vi "clicked_double_circ_trajectory.vi"(0 "ScanModeTS090821Circular2D in":refnum<class "ImagingModeTS090821Circular2D.lvclass">, 1 "clicked points":i32[][](array[numeric]), 7 "error in (no error)":errorcluster) -> (20 "ScanModeTS090821Circular2D out":refnum<class "ImagingModeTS090821Circular2D.lvclass">, 27 "error out":errorcluster)   [LabVIEW 2010, in "ImagingModeTS090821Circular2D.lvclass"]
uses:
  ImagingModeTS090821Circular2D.lvclass
  ImagingModeTS090821Circular2D.lvclass/ImagingModeTS090821Circular2D.ctl
  common/classes/Image/Image/Image.lvclass
  <vilib>/express/express arith-compare/Formula/XNode/ExpressFormulaBlockNode.xnode
  <vilib>/Analysis/BLAS.llb/dnrm2 - Vector 2-Norm (DBL).vi
  <vilib>/Analysis/NI_AALBLAS.lvlib
panel:
  out "rotation angle atan2":dbl
  out "x y centering":dbl[](array[numeric])
  out "circ_offset":dbl
  out "a amplitude":dbl
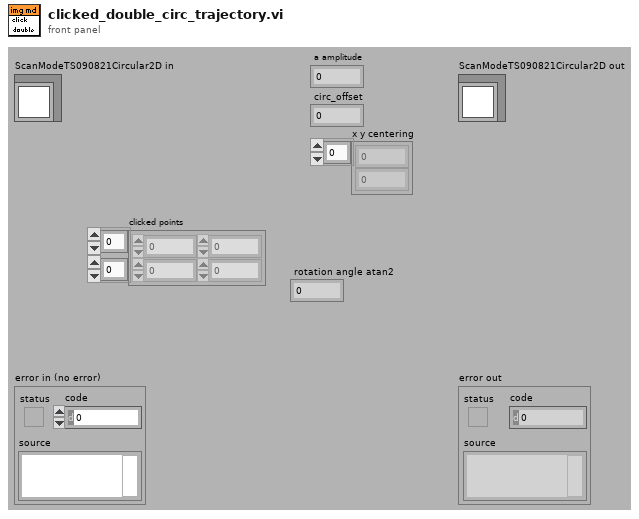
[diagram p1: front panel]
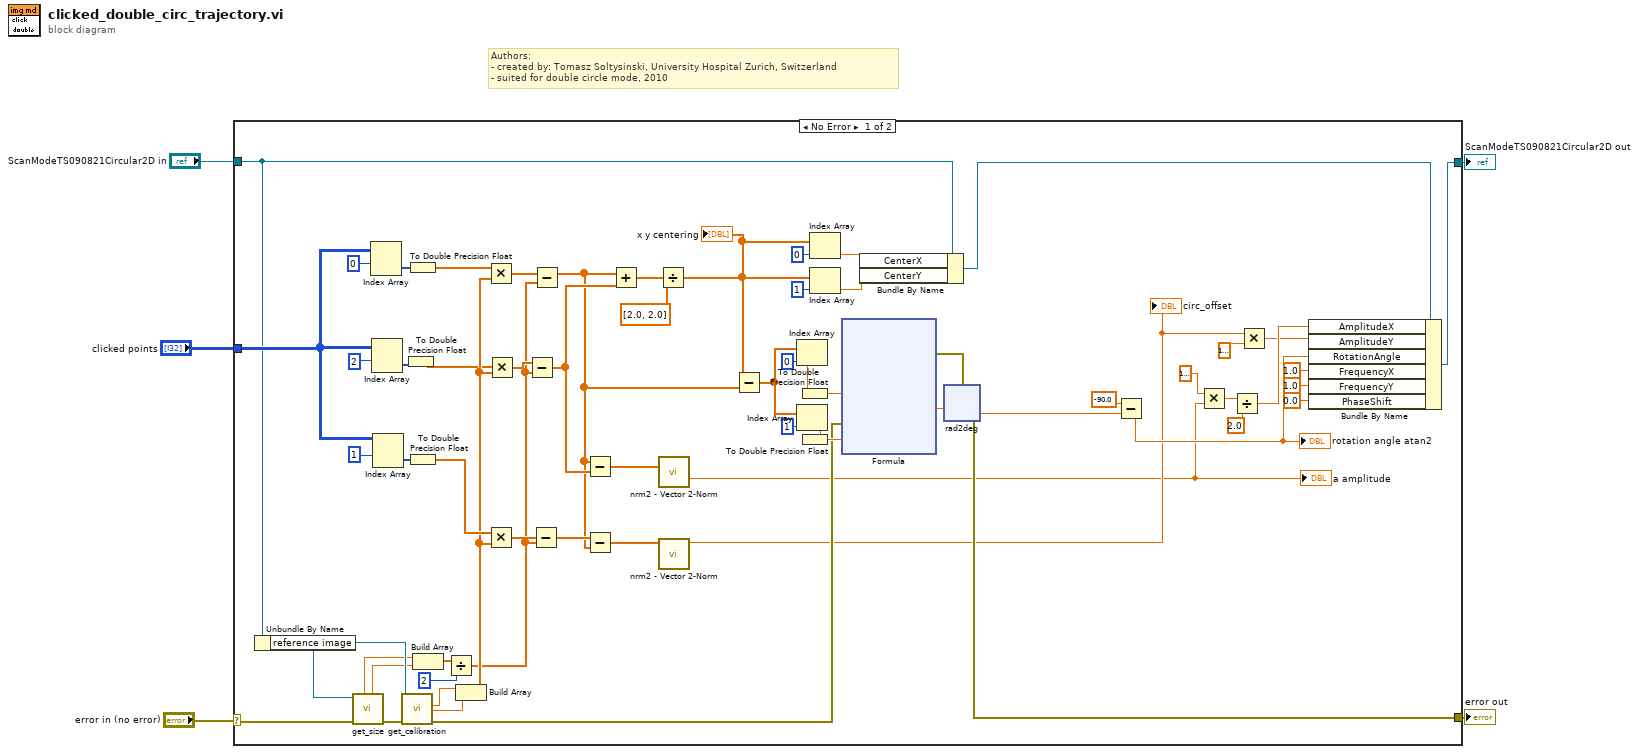
[diagram p0: block diagram]
diagram:
  # "Authors: \n- created by: Tomasz Soltysinski, University Hospital Zurich, Switzerland\n- suited for double circle mode, 2010"
  n1 = case shown="No Error" "error in (no error)" {
    selector: "error in (no error)" -> [w22 w89]
    tunnel: [w9 w89] -> w4
    tunnel: [w55 w88] -> w2
    tunnel: "ScanModeTS090821Circular2D in" -> [w26 w88]
    tunnel: "clicked points" -> [w38 _]
    frame No Error {
      n2 = Unbundle By Name(w26) -> ("reference image"=w20:refnum<class "Image.lvclass">)
      n3 = call-dynamic "get_size.vi"("error in (no error)"=w22, "Image in"=w20) -> ("error out"=w21:errorcluster, "physical size y"=w18:dbl, "physical size x"=w19:dbl)  [unwired: 2 in, 5 out]
      n4 = Index Array(array=w38, index (row)=0 ("disabled index (col)")) -> (element=w37:i32[])  [unwired: 1 in]
      n5 = Index Array(array=w38, index (row)=2 ("disabled index (col)")) -> (element=w36:i32[])  [unwired: 1 in]
      n6 = Index Array(array=w38, index (row)=1 ("disabled index (col)")) -> (element=w35:i32[])  [unwired: 1 in]
      n7 = call "get_calibration.vi"("error in (no error)"=w21, "Image.lvclass in"=w20) -> ("error out"=w25:errorcluster, "y"=w23:dbl, "x"=w24:dbl)  [unwired: 4 in, 3 out]
      n8 = To Double Precision Float(number=w36) -> (double precision float=w29:dbl[])
      n9 = To Double Precision Float(number=w37) -> (double precision float=w28:dbl[])
      n10 = To Double Precision Float(number=w35) -> (double precision float=w31:dbl[])
      n11 = Build Array(w19, w18) -> (w12:dbl[])
      n12 = Divide(x=w12, y=2 ("physical size y")) -> (x/y=w11:dbl[])
      n13 = Build Array(w24, w23) -> (w30:dbl[])
      n14 = Multiply(x=w28, y=w30) -> (x*y=w15:dbl[])
      n15 = Multiply(x=w31, y=w30) -> (x*y=w14:dbl[])
      n16 = Multiply(x=w29, y=w30) -> (x*y=w17:dbl[])
      n17 = Subtract(x=w17, y=w11) -> (x-y=w16:dbl[])
      n18 = Subtract(x=w14, y=w11) -> (x-y=w13:dbl[])
      n19 = Subtract(x=w15, y=w11) -> (x-y=w6:dbl[])
      n20 = Subtract(x=w6, y=w16) -> (x-y=w33:dbl[])
      n21 = Subtract(x=w13, y=w6) -> (x-y=w32:dbl[])
      n22 = Add(x=w6, y=w16) -> (x+y=w34:dbl[])
      n23 = Divide(x=w34, y=dbl[] [2.0, 2.0]) -> (x/y=w27:dbl[])
      "x y centering" <- w27
      n24 = call-poly <vilib>:"nrm2 - Vector 2-Norm.vi"("x"=w33) -> ("dnrm2"=w7:dbl)  [unwired: 9 in, 1 out]
      "a amplitude" <- w7
      n25 = call-poly <vilib>:"nrm2 - Vector 2-Norm.vi"("x"=w32) -> ("dnrm2"=w8:dbl)  [unwired: 9 in, 1 out]
      "circ_offset" <- w8
      n26 = Subtract(x=w27, y=w6) -> (x-y=w52:dbl[])
      n27 = Index Array(array=w52, index=0) -> (element=w51:dbl)
      n28 = Index Array(array=w52, index=1) -> (element=w49:dbl)
      n29 = To Double Precision Float(number=w51) -> (double precision float=w50:dbl)
      n30 = To Double Precision Float(number=w49) -> (double precision float=w48:dbl)
      n31 = Index Array(array=w27, index=0 ("disabled index (col)")) -> (element=w59:dbl)
      n32 = Index Array(array=w27, index=1 ("disabled index (col)")) -> (element=w57:dbl)
      n33 = xnode "Formula"("x"=w50, "error in (no error)"=w25, "y"=w48) -> ("Result"=w46:dbl, "error out"=w44:errorcluster)
      n34 = Bundle By Name(cluster=w26, "CenterX"=w59, "CenterY"=w57) -> (w56:refnum<class "ImagingModeTS090821Circular2D.lvclass">)
      n35 = xnode "rad2deg"("alfa"=w46, "error in (no error)"=w44) -> ("Result"=w45:dbl, "error out"=w9:errorcluster)
      n36 = Subtract(x=-90.0 ("y"), y=w45) -> (x-y=w39:dbl)
      "rotation angle atan2" <- w39
      n37 = Multiply(x=dbl[unit] 1e-06 ("dimension size"), y=w7) -> (x*y=w64:dbl[unit])
      n38 = Divide(x=w64, y=2.0) -> (x/y=w62:dbl[unit])
      n39 = Multiply(x=w8, y=dbl[unit] 1e-06 ("dimension size")) -> (x*y=w40:dbl[unit])
      n40 = Bundle By Name(cluster=w56, "AmplitudeX"=w62, "AmplitudeY"=w40, "RotationAngle"=w39, "FrequencyX"=1.0 ("settings.x frequency"), "FrequencyY"=1.0 ("settings.y frequency"), "PhaseShift"=0.0 ("settings.phase shift")) -> (w55:refnum<class "ImagingModeTS090821Circular2D.lvclass">)
    }
    frame Error {
    }
  }
  "error out" <- w4
  "ScanModeTS090821Circular2D out" <- w2
